vi "Asynchronous Launcher - Keithley DMM.vi"(6 "Worker Alias":string="Fluke DMM", 8 "error in":errorcluster, 9 "Initialization Data":T1, 11 "Fluke DMM in":refnum<class "Keithley DMM.lvclass">) -> (0 "error out":errorcluster, 3 "Fluke DMM out":refnum<class "Keithley DMM.lvclass">)   [LabVIEW 2020, in "Keithley DMM.lvclass"]
doc: "This VI calls a Worker's Launcher VI asynchronously, and returns the Worker's object containing the Worker's Public Accessible data. The returned Worker's object can be used with the Worker's Public API Request VIs from applications external to the Workers application (eg. TestStand).\n---"
uses:
  Keithley DMM.lvclass
  Initialization Data.ctl
  Response Cases.ctl
  Launcher - Fluke DMM.vi
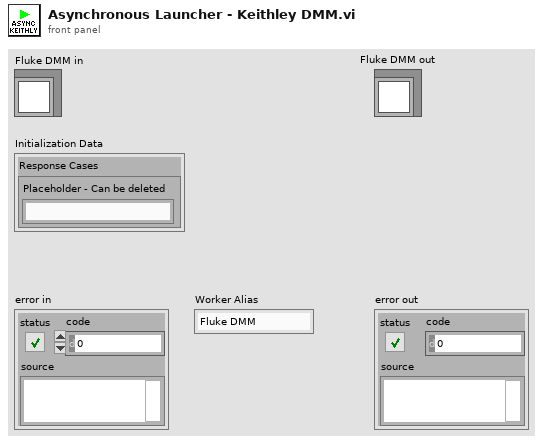
[diagram p1: front panel]
types:
  T1 = typedef "Keithley DMM.lvclass/Initialization Data.ctl" = cluster{"Response Cases":T2}
  T2 = typedef "Keithley DMM.lvclass/Response Cases.ctl" = cluster{"Placeholder - Can be deleted":string}
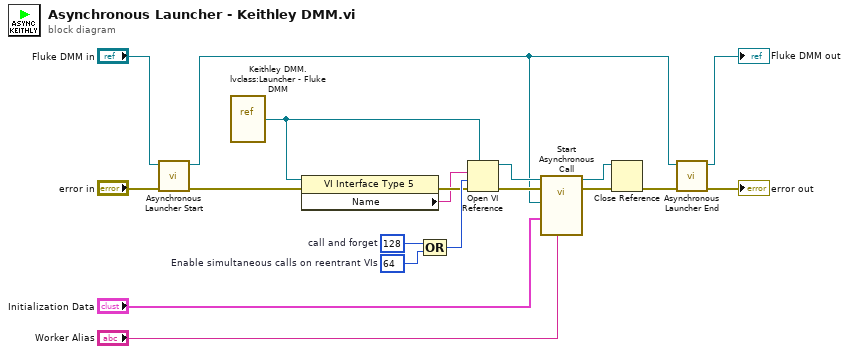
[diagram p0: block diagram]
diagram:
  w18 = 64  # Enable simultaneous calls on reentrant VIs
  w15 = 128  # call and forget
  n1 = call-dynamic "Asynchronous Launcher Start.vi"("error in (no error)"="error in", "Worker in"="Fluke DMM in") -> ("error out"=w19:errorcluster, "Worker out"=w1:refnum<class "Keithley DMM.lvclass">)  [unwired: 8 in]
  n2 = vi-ref "Keithley DMM.lvclass:Launcher - Fluke DMM.vi"() -> (w4:refnum<vi>)
  n3 = property class="VI Interface Type 5"(reference=w4, error in=w19) -> (error out=w13:errorcluster, "Name"=w12:string)  [unwired: 1 out]
  n4 = Compound Arithmetic op=OR(w15, w18) -> (w16:i32)
  n5 = Open VI Reference(type specifier VI Refnum (for type only)=w4, vi path=w12, options=w16, error in (no error)=w13) -> (vi reference=w17:refnum<vi>, error out=w11:errorcluster)  [unwired: 2 in]
  n6 = call-by-ref "Start Asynchronous Call"(reference=w17, error in=w11, "Worker Alias"="Worker Alias", "Initialization Data"="Initialization Data", "Fluke DMM in"=w1) -> (reference out=w9:refnum<vi>, error out=w10:errorcluster)  [unwired: 8 in, 1 out]
  n7 = Close Reference(reference=w9, error in (no error)=w10) -> (error out=w14:errorcluster)
  n8 = call-dynamic "Asynchronous Launcher End.vi"("error in (no error)"=w14, "Worker in"=w1) -> ("error out"=→"error out":errorcluster, "Worker out"=→"Fluke DMM out":refnum<class "Keithley DMM.lvclass">)  [unwired: 8 in]
